vi "ChangeUnit.vi"(0 "change in":dbl, 1 "unit in":string) -> (2 "change out":string, 3 "DataOut":string, 4 "UintOut":string)   [LabVIEW 2018]
panel:
  out "change unit":string
  out "change out":dbl
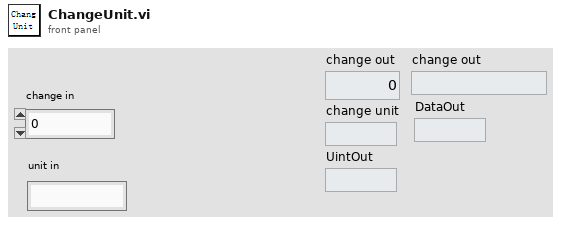
[diagram p1: front panel]
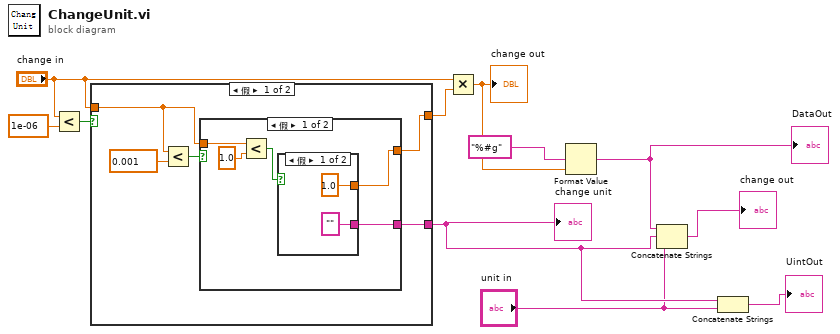
[diagram p0: block diagram]
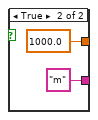
[diagram p2: hidden frame]
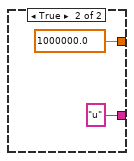
[diagram p3: hidden frame]
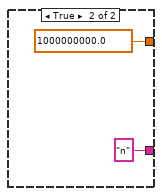
[diagram p4: hidden frame]
diagram:
  n1 = Less?(x="change in", y=1e-06) -> (x < y?=w10:bool)
  n2 = case shown="假" w10 {
    tunnel: [w13 "n"] -> w3
    tunnel: [w14 1000000000.0 ("y")] -> w9
    tunnel: "change in" -> [w12 _]
    frame False {
      n3 = Less?(x=w12, y=0.001) -> (x < y?=w15:bool)
      n4 = case shown="假" w15 {
        tunnel: [w17 1000000.0 ("y")] -> w14
        tunnel: [w19 "u"] -> w13
        tunnel: w12 -> [w21 _]
        frame False {
          n5 = Less?(x=w21, y=1.0) -> (x < y?=w18:bool)
          n6 = case shown="假" w18 {
            tunnel: ["" "m"] -> w19
            tunnel: [1.0 ("y") 1000.0 ("y")] -> w17
            frame False {
            }
            frame True {
            }
          }
        }
        frame True {
        }
      }
    }
    frame True {
    }
  }
  "change unit" <- w3
  n7 = Multiply(x="change in", y=w9) -> (x*y=w7:dbl)
  "change out" <- w7
  n8 = Format Value(format string="%#g" ("字符串(\"\")"), value (0)=w7) -> (output string=w5:string)  [unwired: 1 in]
  "DataOut" <- w5
  n9 = Concatenate Strings(w5, w3, "unit in") -> (→"change out":string)
  n10 = Concatenate Strings(w3, "unit in") -> (→"UintOut":string)
